vi "Register Open Sequences.vi"(8 "Error In":errorcluster, 10 "Application Manager In":refnum<k7>, 11 "Register In":map{string, T1}(c390)) -> (0 "Error Out":errorcluster, 3 "Register Out":map{string, T1}(c390))   [LabVIEW 2021, in "Seq Edit Quick Drop.lvlib"]
uses:
  Seq Edit Quick Drop.lvlib
  Register Item.ctl
  ea29a42a-2546-4133-91d3-0e7f559e21e7.vi
  Compare IDs.vi/1e67f69e-a106-45ae-a325-7203d080973c.vi
  Compare IDs.vi/67f33a7c-9d8a-4da2-8438-0c57403dbbc6.vi
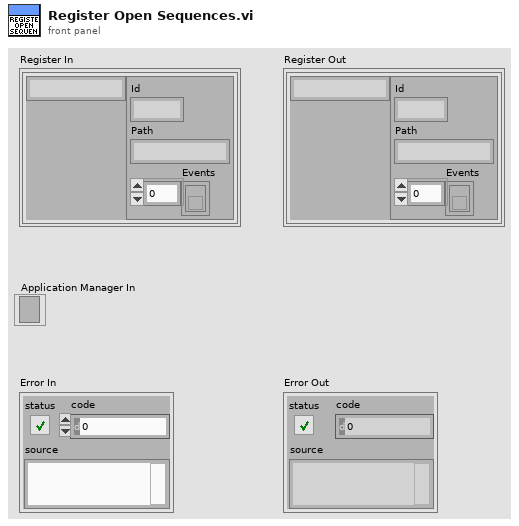
[diagram p1: front panel]
types:
  T1 = typedef "Seq Edit Quick Drop.lvlib/Register Item.ctl" = cluster{"Id":i32, "Path":string, "Events":refnum<k27>[]}
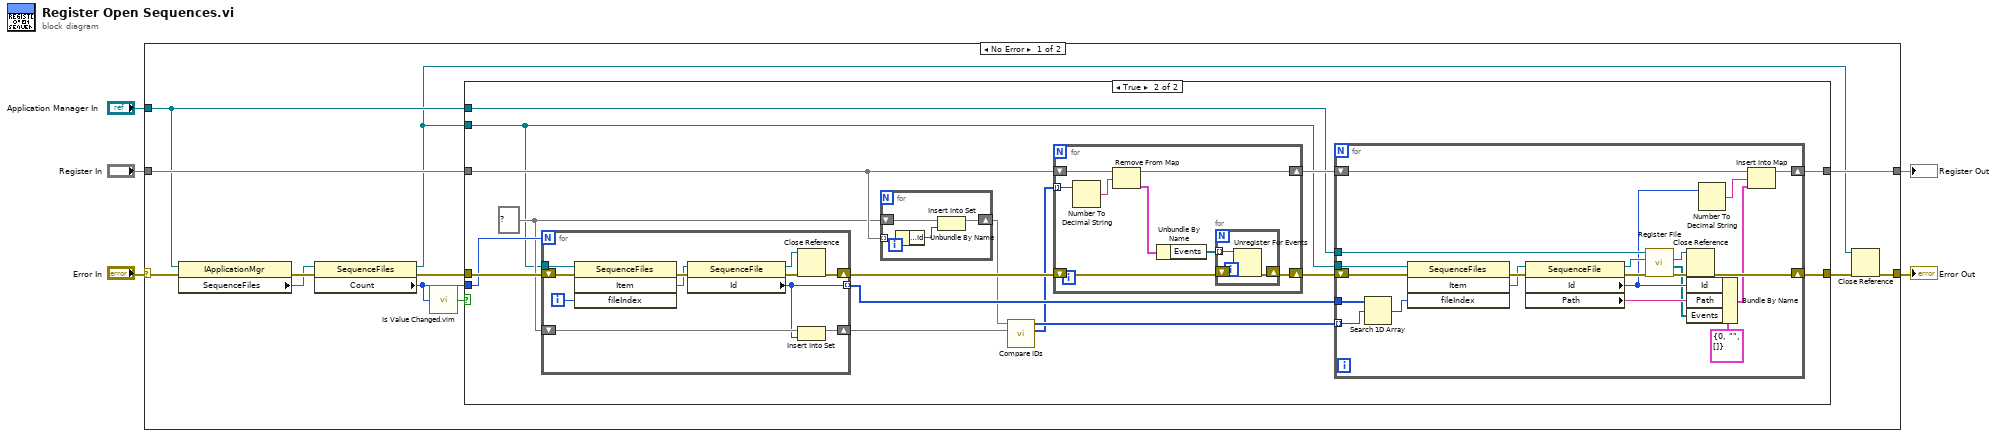
[diagram p0: block diagram]
diagram:
  n1 = case shown="No Error" "Error In" {
    selector: "Error In" -> [w10 w84]
    tunnel: "Application Manager In" -> [w9 _]
    tunnel: "Register In" -> [w15 w83]
    tunnel: [w12 w83] -> w1
    tunnel: [w7 w84] -> w3
    frame No Error {
      n2 = property class="IApplicationMgr"(reference=w9, error in=w10) -> (error out=w17:errorcluster, "SequenceFiles"=w8:refnum<k7>)  [unwired: 1 out]
      n3 = property class="SequenceFiles"(reference=w8, error in=w17) -> (reference out=w6:refnum<k7>, error out=w14:errorcluster, "Count"=w13:i32)
      n4 = call "Is Value Changed.vim"("value"=w13) -> ("changed or first call?"=w16:bool)
      n5 = case shown="True" w16 {
        tunnel: w6 -> [_ w22]
        tunnel: w9 -> [_ w28]
        tunnel: w15 -> [w19 w27]
        tunnel: w14 -> [w18 w32]
        tunnel: w13 -> [_ w26]
        tunnel: [w19 w21] -> w12
        tunnel: [w18 w20] -> w11
        frame False {
        }
        frame True {
          w25 = set{i32} {} ("Size: 0")
          n6 = for {
            N: w26 -> [_]
            tunnel: w22 -> [w60]
            shift-right: [w55] -> w33
            shift-left: w32 -> [w54]
            shift-right: [w53] -> w31
            shift-left: w25 -> [w52]
            tunnel: [w51] -> w30 mode=indexing
            i -> [w59]
            n7 = invoke class="SequenceFiles" method="Item"(reference=w60, error in=w54, "fileIndex"=w59) -> (error out=w61:errorcluster, "Item"=w58:refnum<k7>)  [unwired: 1 in, 2 out]
            n8 = property class="SequenceFile"(reference=w58, error in=w61) -> (reference out=w57:refnum<k7>, error out=w56:errorcluster, "Id"=w51:i32)
            n9 = Close Reference(reference=w57, error in (no error)=w56) -> (error out=w55:errorcluster)
            n10 = Insert Into Set(10:w51, 11:w52) -> (3:w53:set{i32})  [unwired: 1 out]
          }
          n11 = for {
            tunnel: w27 -> [w39] mode=indexing
            shift-right: [w37] -> w23
            shift-left: w25 -> [w38]
            n12 = Unbundle By Name(w39) -> ("Register Item.Id"=w36:i32)
            n13 = Insert Into Set(10:w36, 11:w38) -> (3:w37:set{i32})  [unwired: 1 out]
          }
          n14 = call "Compare IDs.vi"("New IDs"=w31, "Current IDs"=w23) -> ("Removed IDs"=w24:i32[], "Added IDs"=w29:i32[])  [unwired: 7 in, 1 out]
          n15 = for {
            tunnel: w24 -> [w46] mode=indexing
            shift-right: [w44] -> w35
            shift-left: w27 -> [w47]
            shift-right: [w40] -> w34
            shift-left: w33 -> [w41]
            n16 = Number To Decimal String(number=w46) -> (decimal integer string=w45:string)  [unwired: 1 in]
            n17 = Remove From Map(10:w45, 11:w47) -> (1:w43:T1, 3:w44:map{string, T1})  [unwired: 1 out]
            n18 = Unbundle By Name(w43) -> ("Events"=w42:refnum<k27>[])
            n19 = for {
              tunnel: w42 -> [w50] mode=indexing
              shift-right: [w48] -> w40
              shift-left: w41 -> [w49]
              n20 = Unregister For Events(event registration refnum=w50, error in=w49) -> (error out=w48:errorcluster)
            }
          }
          n21 = for {
            tunnel: w30 -> [w80]
            tunnel: w29 -> [w79] mode=indexing
            tunnel: w22 -> [w73]
            tunnel: w28 -> [w72]
            shift-right: [w70] -> w20
            shift-left: w34 -> [w71]
            shift-right: [w62] -> w21
            shift-left: w35 -> [w63]
            n22 = Search 1D Array(1D array=w80, element=w79) -> (index of element=w78:i32)  [unwired: 1 in]
            n23 = invoke class="SequenceFiles" method="Item"(reference=w73, error in=w71, "fileIndex"=w78) -> (error out=w77:errorcluster, "Item"=w76:refnum<k7>)  [unwired: 1 in, 2 out]
            n24 = property class="SequenceFile"(reference=w76, error in=w77) -> (reference out=w69:refnum<k7>, error out=w74:errorcluster, "Id"=w68:i32, "Path"=w75:string)
            n25 = call "Register File.vi"("Error In"=w74, "Sequence File In"=w69, "Application Manager In"=w72) -> ("Error out"=w81:errorcluster, "Events"=w67:refnum<k27>[], "Sequence File Out"=w66:refnum<k7>)  [unwired: 5 in, 1 out]
            n26 = Close Reference(reference=w66, error in (no error)=w81) -> (error out=w70:errorcluster)
            n27 = Bundle By Name(cluster=T1 {"Id"=0, "Path"="", "Events"=[]} ("Register Item"), "Id"=w68, "Path"=w75, "Events"=w67) -> (w64:T1)
            n28 = Number To Decimal String(number=w68) -> (decimal integer string=w82:string)  [unwired: 1 in]
            n29 = Insert Into Map(map in=w63, key=w82, value=w64) -> (map out=w62:map{string, T1})  [unwired: 2 out]
          }
        }
      }
      n30 = Close Reference(reference=w6, error in (no error)=w11) -> (error out=w7:errorcluster)
    }
    frame Error {
    }
  }
  "Error Out" <- w3
  "Register Out" <- w1
